vi "SubVI_Decoder_002.vi"(1 "Cluster templates":cluster{i32[], i32[][]}, 2 "Object IMG Cluster":T1, 3 "Decoder Parameters":T2) -> (0 "Results, dissimilarity, pixs":cluster{"Result":string, "Dissimilarity":dbl[]})   [LabVIEW 2018]
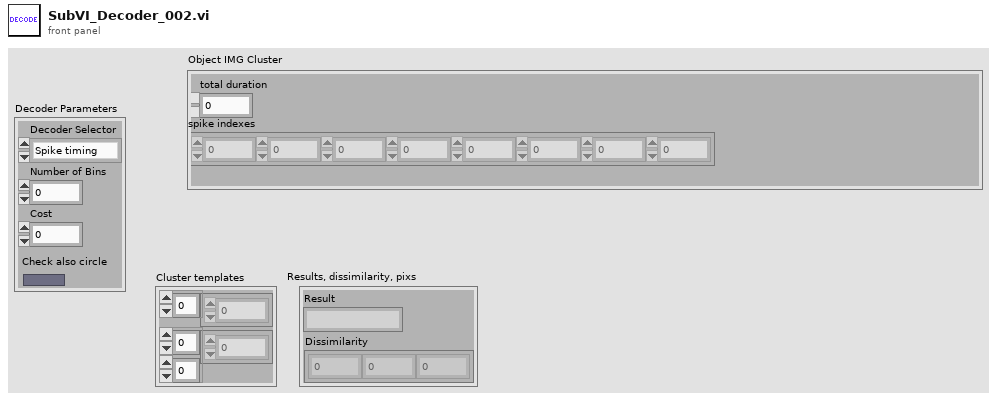
[diagram p1: front panel]
types:
  T1 = cluster{"total duration":i32, "spike indexes":i32[]}
  T2 = cluster{"Decoder Selector":enum16{"Spike timing", "Spike counting", "Victor Purpura"}, "Number of Bins":i32, "Cost":dbl, "Check also circle":bool}
  T3 = enum16{"Spike timing", "Spike counting", "Victor Purpura"}
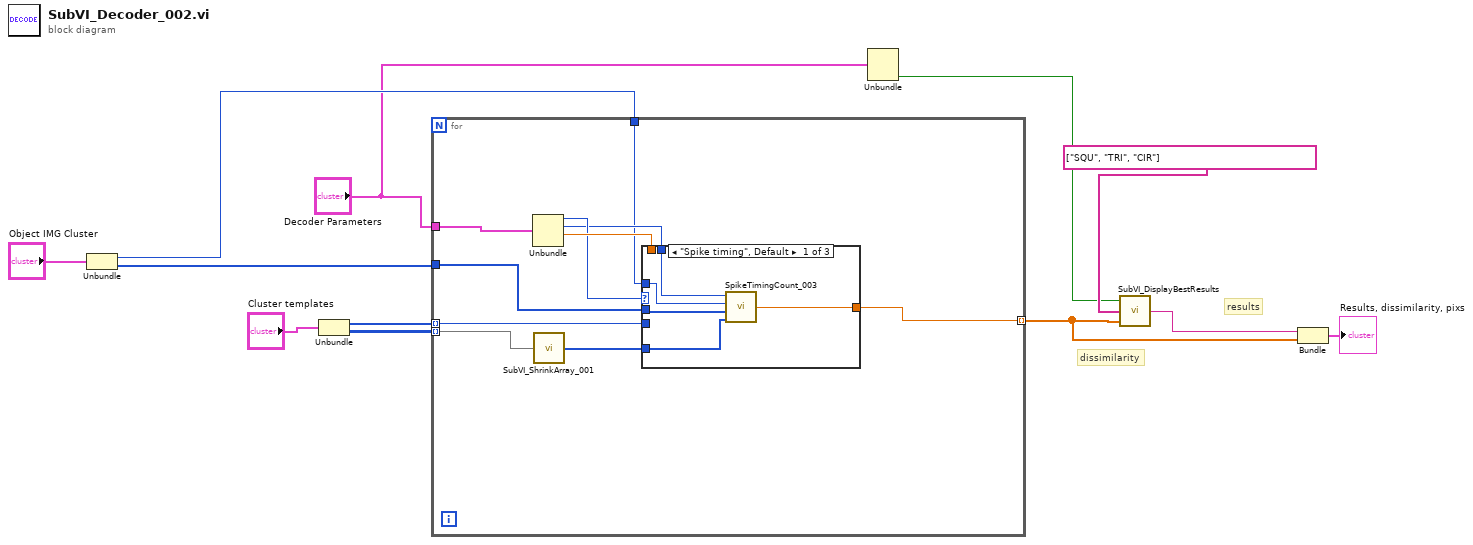
[diagram p0: block diagram]
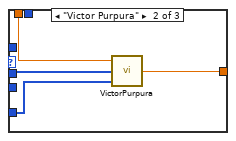
[diagram p2: hidden frame]
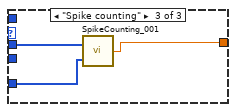
[diagram p3: hidden frame]
diagram:
  # "dissimilarity"
  # "results"
  n1 = Unbundle("Object IMG Cluster") -> ("total duration"=w8:i32, "spike indexes"=w7:i32[])
  n2 = Unbundle("Cluster templates") -> (w11:i32[], w10:i32[][])
  n3 = for {
    tunnel: w7 -> [w22]
    tunnel: "Decoder Parameters" -> [w18]
    tunnel: w11 -> [w16] mode=indexing
    tunnel: w10 -> [w14] mode=indexing
    tunnel: [w17] -> w4 mode=indexing
    tunnel: w8 -> [w15]
    n4 = Unbundle(w18) -> ("Decoder Selector"=w20:T3, "Number of Bins"=w19:i32, "Cost"=w21:dbl)  [unwired: 1 out]
    n5 = call "SubVI_ShrinkArray_001.vi"("Input Array"=w14) -> ("Output Array"=w13:i32[])
    n6 = case shown="\"Spike timing\", Default" w20 {
      tunnel: w19 -> [w27 _ _]
      tunnel: w22 -> [w26 w29 w34]
      tunnel: w21 -> [_ w30 _]
      tunnel: w16 -> [_ _ _]
      tunnel: [w23 w31 w32] -> w17
      tunnel: w13 -> [w25 w28 w33]
      tunnel: w15 -> [w24 _ _]
      frame "Spike timing", Default {
        n7 = call "SpikeTimingCount_003.vi"("template"=w25, "Test object"=w26, "Total Duration"=w24, "Number of Bins"=w27) -> ("Dissimilarity"=w23:dbl)
      }
      frame "Victor Purpura" {
        n8 = call "VictorPurpura.vi"("template"=w28, "Test Object"=w29, "Cost"=w30) -> ("dissimilarity"=w31:dbl)
      }
      frame "Spike counting" {
        n9 = call "SpikeCounting_001.vi"("Template"=w33, "Test object"=w34) -> ("dissimiliarity"=w32:dbl)
      }
    }
  }
  n10 = Unbundle("Decoder Parameters") -> ("Check also circle"=w2:bool)  [unwired: 3 out]
  n11 = call "SubVI_DisplayBestResults.vi"("Dissimilarity values (in)"=w4, "Objects to compare it to"=string[] ["SQU", "TRI", "CIR"], "Check also circle"=w2) -> ("Result"=w1:string)
  n12 = Bundle("Result"=w1, w4) -> (→"Results, dissimilarity, pixs":cluster{"Result":string, dbl[]})  [unwired: 1 in]
